vi "SubVI_Identificador_de_objetos_alterado.vi"(8 "error in (no error)":errorcluster, 9 "ROI Detecção":T3 {"Contours"."Type" items=["No Selection", "Point", "Line", "Rectangle", "Oval", "Polygon", "Free", "Annulus", "Unused2", "Unused3", "Broken Line", "Free Hand Line", "Rotated Rectangle"]}, 10 "ROI Esteira":T3 {"Contours"."Type" items=["No Selection", "Point", "Line", "Rectangle", "Oval", "Polygon", "Free", "Annulus", "Unused2", "Unused3", "Broken Line", "Free Hand Line", "Rotated Rectangle"]}, 11 "Session In":T2) -> (0 "error out":errorcluster, 3 "Objeto Identificado":bool)   [LabVIEW 2017]
uses:
  <vilib>/userdefined/High Color/IMAQdx.ctl
  <vilib>/vision/driver/IMAQdx.llb/IMAQdx Buffer Number Mode.ctl
  <vilib>/vision/driver/NI_Vision_Acquisition_Software.lvlib
  <vilib>/vision/NI_Vision_Development_Module.lvlib
panel:
  out "Imagem Original":T1(plugin-control)
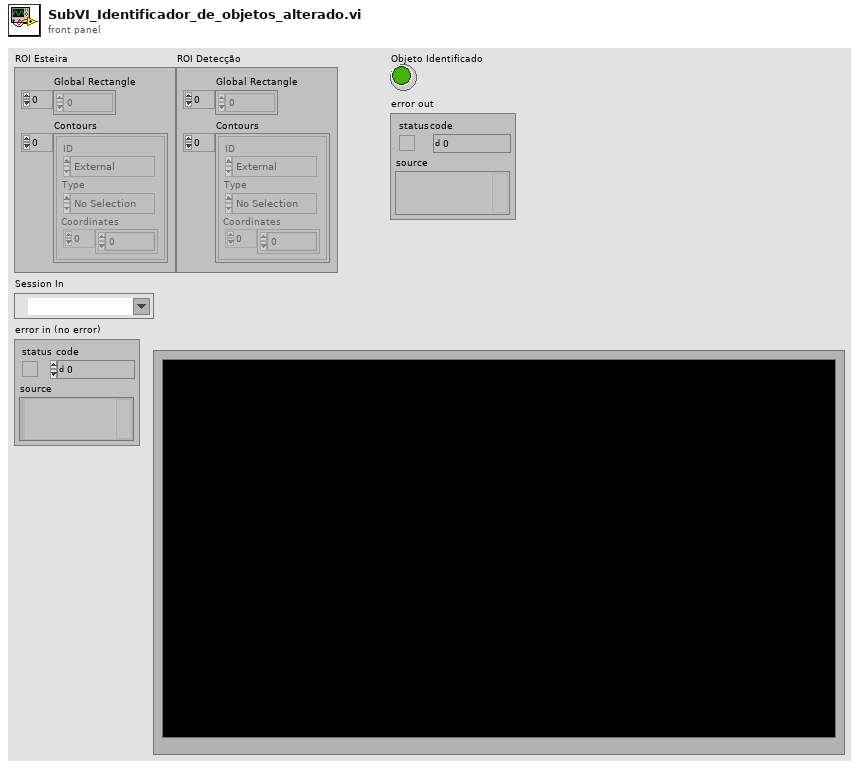
[diagram p1: front panel]
types:
  T1 = typedef "IMAQ Image.ctl" = refnum<image>
  T2 = typedef "IMAQdx.ctl" = refnum<k21>
  T3 = cluster{"Global Rectangle":i32[], "Contours":cluster{"ID":enum32{"External", "Internal"}, "Type":u32, "Coordinates":i32[]}[]}
  T4 = cluster{"Objects":u16, "Threshold":i32, "Reject Border":bool, "Fill Holes":bool, "Min Object Size":bool, "Min Size":i32, "Max Object Size":bool, "Max Size":i32, "Show Search Area":bool, "Show Center":bool, "Show Bounding Box":bool}
  T5 = typedef "NI_Vision_Acquisition_Software.lvlib/IMAQdx Buffer Number Mode.ctl" = enum32{"Next", "Last", "Buffer Number", "Every", "Last New"}
  T6 = typedef "Image Type" = u32
  T7 = typedef "IMAQ Rectangle" = cluster{"Left":i32, "Top":i32, "Right":i32, "Bottom":i32, "Rotation":dbl}
  T8 = cluster{"Object Center":cluster{"X":sgl, "Y":sgl}, "Bounding Box":cluster{"X Left":i32, "Y Top":i32, "X Right":i32, "Y Bottom":i32}, "Area":sgl, "Orientation":sgl, "Aspect Ratio":sgl, "Nb Holes":i32}[]
  T9 = cluster{"Object Center":cluster{"X":sgl, "Y":sgl}, "Bounding Box":cluster{"X Left":i32, "Y Top":i32, "X Right":i32, "Y Bottom":i32}, "Area":sgl, "Orientation":sgl, "Aspect Ratio":sgl, "Nb Holes":i32}
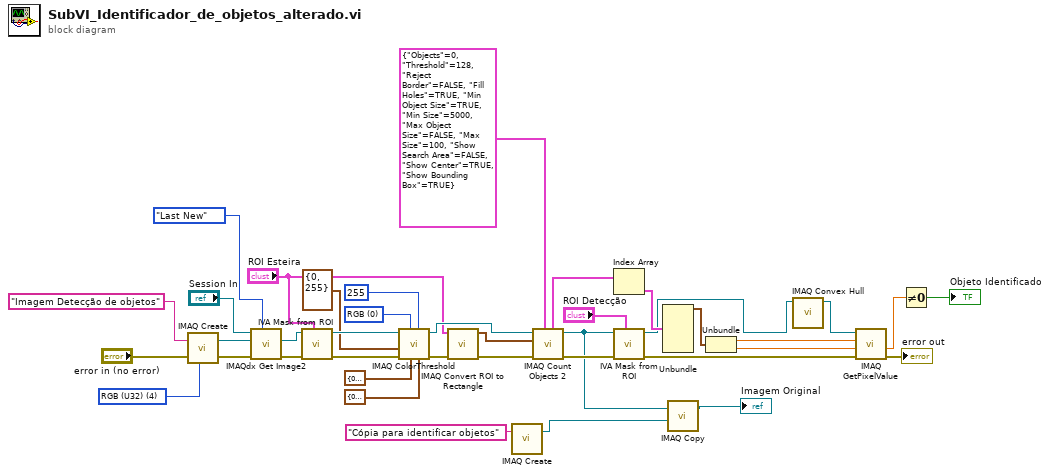
[diagram p0: block diagram]
diagram:
  w32 = u16 0 items=["RGB", "HSL", "HSV", "HSI"] ("Color Mode")
  w38 = T6 4 items=["Grayscale (U8)", "Grayscale (I16)", "Grayscale (SGL)", "Complex (CSG)", "RGB (U32)", "HSL (U32)", "RGB (U64)", "Grayscale (U16)"] ("Image Type")
  n1 = call "IMAQ Create"("Image Name"="Imagem Detecção de objetos", "Image Type"=w38, "error in (no error)"="error in (no error)") -> ("New Image"=w36:T1, "error out"=w35:errorcluster)  [unwired: 2 in]
  n2 = call <vilib>:"IMAQdx Get Image2.vi"("Buffer Number Mode (Next)"=IMAQdx_Buffer_Number_Mode."Last New", "error in"=w35, "Image In"=w36, "Session In"="Session In") -> ("error out"=w13:errorcluster, "Image Out"=w34:T1)  [unwired: 4 in, 2 out]
  n3 = call <vilib>:"IVA Mask from ROI.vi"("ROI Descriptor"="ROI Esteira", "error in (no error)"=w13, "Image Src"=w34) -> ("error out"=w12:errorcluster, "Image Out"=w33:T1)  [unwired: 2 in, 5 out]
  n4 = call "IMAQ ColorThreshold"("Blue or Luma or Val or Inten Range"=cluster{"Lower value":i32, "Upper value":i32} {"Lower value"=0, "Upper value"=150}, "Replace Value"=255, "Green or Sat Range"=cluster{"Lower value":i32, "Upper value":i32} {"Lower value"=0, "Upper value"=255}, "Color Mode"=w32, "error in (no error)"=w12, "Red or Hue Range"=cluster{"Lower value":i32, "Upper value":i32} {"Lower value"=0, "Upper value"=255}, "Image Src"=w33) -> ("error out"=w11:errorcluster, "Image Dst Out"=w25:T1)  [unwired: 1 in, 2 out]
  n5 = call "IMAQ Convert ROI to Rectangle"("error in (no error)"=w11, "ROI Descriptor"="ROI Esteira") -> ("error out"=w10:errorcluster, "Rectangle"=w26:T7)  [unwired: 7 in]
  n6 = call "IMAQ Create"("Image Name"="Cópia para identificar objetos") -> ("New Image"=w2:T1)  [unwired: 4 in, 1 out]
  n7 = call "IMAQ Count Objects 2"("Settings"=T4 {"Objects"=0, "Threshold"=128, "Reject Border"=FALSE, "Fill Holes"=TRUE, "Min Object Size"=TRUE, "Min Size"=5000, "Max Object Size"=FALSE, "Max Size"=100, "Show Search Area"=FALSE, "Show Center"=TRUE, "Show Bounding Box"=TRUE}, "error in (no error)"=w10, "Search Rect (entire image)"=w26, "Image"=w25) -> ("error out"=w9:errorcluster, "Image Out"=w1:T1, "Objects"=w24:T8)  [unwired: 3 in, 2 out]
  n8 = Index Array(array=w24) -> (element=w23:T9)  [unwired: 1 in]
  n9 = call <vilib>:"IVA Mask from ROI.vi"("ROI Descriptor"="ROI Detecção", "error in (no error)"=w9, "Image Src"=w1) -> ("error out"=w8:errorcluster, "Image Out"=w6:T1)  [unwired: 2 in, 5 out]
  n10 = Unbundle(w23) -> ("Object Center"=w7:cluster{"X":sgl, "Y":sgl})  [unwired: 5 out]
  n11 = call "IMAQ Copy"("Image Dst"=w2, "Image Src"=w1) -> ("Image Dst Out"=→"Imagem Original":T1)  [unwired: 4 in, 1 out]
  n12 = Unbundle(w7) -> ("X"=w22:sgl, "Y"=w21:sgl)
  n13 = call "IMAQ Convex Hull"("Image Src"=w6) -> ("Image Dst Out"=w5:T1)  [unwired: 9 in, 1 out]
  n14 = call "IMAQ GetPixelValue"("Image"=w5, "X Coordinate"=w22, "Y Coordinate"=w21, "error in (no error)"=w8) -> ("Pixel Value (Float)"=w20:sgl, "error out"=→"error out":errorcluster)  [unwired: 2 in, 3 out]
  n15 = Not Equal To 0?(x=w20) -> (x != 0?=→"Objeto Identificado":bool)
